vi "Example Graph.vi"() -> ()   [LabVIEW 2013]
uses:
  C:/tf/play/labview/Tinkerforge.dll
  Tinkerforge.dll
panel:
  in  "stop":bool
  out "graph":sgl[](graph)
  in  "uid":string="kpV"
  in  "port":i32=4223
  in  "host":string="localhost"
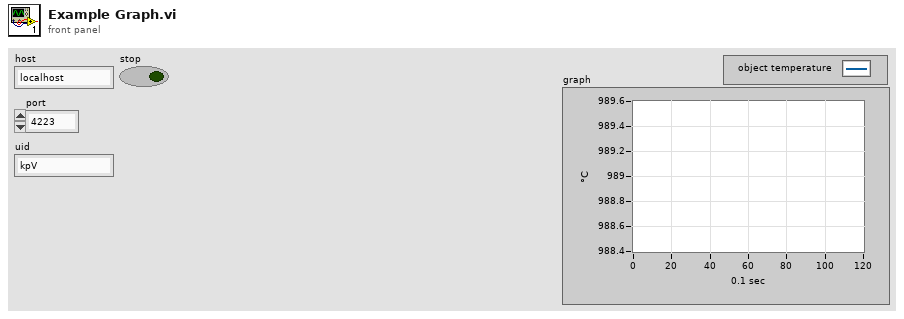
[diagram p1: front panel]
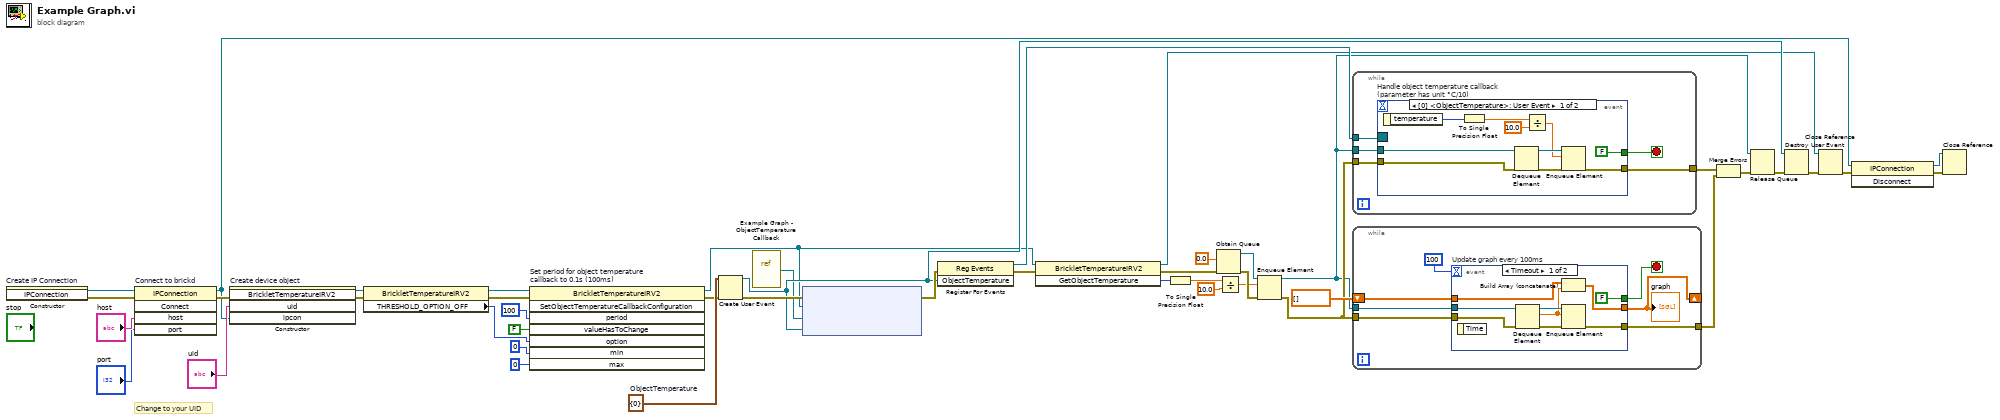
[diagram p0: block diagram]
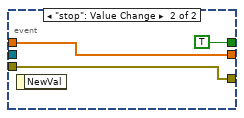
[diagram p2: hidden frame]
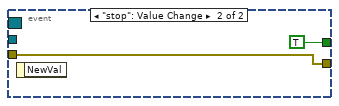
[diagram p3: hidden frame]
diagram:
  w31 = cluster{"temperature":i16} {"temperature"=0}  # ObjectTemperature
  # "Change to your UID"
  n1 = constructor on="Create IP Connection" class="IPConnection"() -> (reference out=w45:refnum<k24>, error out=w18:errorcluster)  [unwired: 3 in, 1 out]
  n2 = invoke on="Connect to brickd" class="IPConnection" method="Connect"(reference=w45, error in=w18, "host"="host", "port"="port") -> (reference out=w38:refnum<k24>, error out=w41:errorcluster)  [unwired: 1 in, 3 out]
  n3 = constructor on="Create device object" class="BrickletTemperatureIRV2"(error in=w41, "uid"="uid", "ipcon"=w38) -> (reference out=w5:refnum<k24>, error out=w4:errorcluster)  [unwired: 2 in, 3 out]
  n4 = property class="BrickletTemperatureIRV2"(reference=w5, error in=w4) -> (reference out=w2:refnum<k24>, error out=w3:errorcluster, "THRESHOLD_OPTION_OFF"=w1:u16)
  n5 = invoke on="Set period for object temperature\ncallback to 0.1s (100ms)" class="BrickletTemperatureIRV2" method="SetObjectTemperatureCallbackConfiguration"(reference=w2, error in=w3, "period"=i64 100, "valueHasToChange"=FALSE, "option"=w1, "min"=i16 0, "max"=i16 0) -> (reference out=w15:refnum<k24>, error out=w30:errorcluster)  [unwired: 1 in, 6 out]
  n6 = Create User Event(user event datatype=w31, error in=w30) -> (user event=w33:refnum<user-event>, error out=w36:errorcluster)
  n7 = vi-ref "Example Graph - ObjectTemperature Callback.vi"() -> ("vi reference"=w9:refnum<vi>)
  n8 = node ("Register Event Callback")(w36, w15, w9, w33) -> (w35:errorcluster)  [unwired: 1 in, 1 out]
  n9 = register-events(error in=w35, w33) -> (reference out=w34:refnum<event-registration>, error out=w17:errorcluster)  [unwired: 1 in]
  n10 = invoke class="BrickletTemperatureIRV2" method="GetObjectTemperature"(reference=w15, error in=w17) -> (reference out=w14:refnum<k24>, error out=w16:errorcluster, "GetObjectTemperature"=w10:i16)  [unwired: 1 in]
  n11 = To Single Precision Float(number=w10) -> (single precision float=w13:sgl)
  n12 = Obtain Queue(element data type=sgl 0.0, error in (no error)=w16) -> (queue out=w22:refnum<queue>, error out=w24:errorcluster)  [unwired: 3 in, 1 out]
  n13 = Divide(x=w13, y=sgl 10.0) -> (x/y=w11:sgl)
  n14 = Enqueue Element(queue=w22, element=w11, error in (no error)=w24) -> (queue out=w19:refnum<queue>, error out=w23:errorcluster)  [unwired: 1 in, 1 out]
  n15 = while {
    tunnel: w34 -> [w50]
    tunnel: [w48] -> w27
    tunnel: w23 -> [w49]
    tunnel: w19 -> [w47]
    stop <- w46 stop-if-true
    n16 = event "Handle object temperature callback (parameter has unit °C/10)" shown="[0] <ObjectTemperature>: User Event" {
      selector: w50 -> [_ _]
      dyn-events: _ -> [_ _]
      timeout: _ -> [_ _]
      tunnel: w49 -> [w57 w61]
      tunnel: [w55 w61] -> w48
      tunnel: w47 -> [w54 _]
      tunnel: [FALSE TRUE] -> w46
      event User Event {
        n17 = event-data() -> ("temperature"=w58:i16)  [unwired: 1 in]
        n18 = To Single Precision Float(number=w58) -> (single precision float=w59:sgl)
        n19 = Dequeue Element(queue=w54, error in (no error)=w57) -> (queue out=w53:refnum<queue>, error out=w56:errorcluster)  [unwired: 1 in, 2 out]
        n20 = Divide(x=w59, y=sgl 10.0) -> (x/y=w52:sgl)
        n21 = Enqueue Element(queue=w53, element=w52, error in (no error)=w56) -> (error out=w55:errorcluster)  [unwired: 1 in, 2 out]
      }
      event "stop": Value Change {
        n22 = event-data() -> ()  [unwired: 1 in, 1 out]
      }
    }
  }
  n23 = while {
    tunnel: [w65] -> w28
    tunnel: w23 -> [w66]
    shift-right: [w67] -> _
    shift-left: sgl[] [] -> [w68]
    tunnel: w19 -> [w64]
    stop <- w63 stop-if-true
    n24 = event "Update graph every 100ms" shown="[0] Timeout" {
      selector: _ -> [_ _]
      dyn-events: _ -> [_ _]
      timeout: 100 -> [_ _]
      tunnel: [w78 w80] -> w67
      tunnel: w68 -> [w71 w80]
      tunnel: w66 -> [w77 w79]
      tunnel: [w74 w79] -> w65
      tunnel: w64 -> [w76 _]
      tunnel: [FALSE TRUE] -> w63
      event Timeout {
        n25 = event-data() -> ()  [unwired: 1 in, 1 out]
        n26 = Dequeue Element(queue=w76, error in (no error)=w77) -> (queue out=w73:refnum<queue>, element=w72:sgl, error out=w75:errorcluster)  [unwired: 1 in, 1 out]
        n27 = Build Array (concatenate)(w71, w72) -> (w78:sgl[])
        n28 = Enqueue Element(queue=w73, element=w72, error in (no error)=w75) -> (error out=w74:errorcluster)  [unwired: 1 in, 2 out]
      }
      event "stop": Value Change {
        n29 = event-data() -> ()  [unwired: 1 in, 1 out]
      }
    }
    "graph" <- w67
  }
  n30 = Merge Errors(w27, w28) -> (w21:errorcluster)
  n31 = Release Queue(queue=w19, error in (no error)=w21) -> (error out=w20:errorcluster)  [unwired: 1 in, 2 out]
  n32 = Destroy User Event(user event=w33, error in=w20) -> (error out=w32:errorcluster)
  n33 = Close Reference(reference=w14, error in (no error)=w32) -> (error out=w40:errorcluster)
  n34 = invoke class="IPConnection" method="Disconnect"(reference=w38, error in=w40) -> (reference out=w37:refnum<k24>, error out=w39:errorcluster)  [unwired: 1 in, 1 out]
  n35 = Close Reference(reference=w37, error in (no error)=w39) -> ()  [unwired: 1 out]
